vi "PasarArray_A_Signal.vi"(11 "subarray":u16[](array[numeric])) -> (3 "Waveform":waveform(dbl))   [LabVIEW 2024]
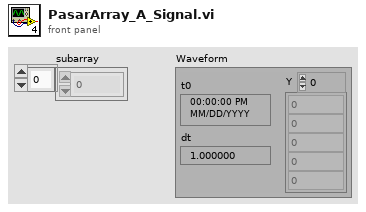
[diagram p1: front panel]
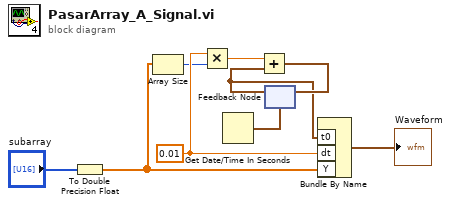
[diagram p0: block diagram]
diagram:
  w6 = 0.01
  n1 = To Double Precision Float(number="subarray") -> (double precision float=w4:dbl[])
  n2 = Array Size(array=w4) -> (size(s)=w5:i32)
  n3 = Multiply(x=w6, y=w5) -> (x*y=w7:dbl)
  n4 = Get Date/Time In Seconds() -> (seconds since 1Jan1904=w3:timestamp)
  n5 = feedback #1(w3) -> (w8:timestamp)
  n6 = Add(x=w7, y=w8) -> (x+y=w9:timestamp)
  n7 = feedback-in #1(w9) -> ()
  n8 = Bundle By Name("t0"=w8, "dt"=w6, "Y"=w4) -> (→"Waveform":waveform(dbl))  [unwired: 1 in]
